vi "Periodic Tasks.vi"(8 "error in":errorcluster) -> ()   [LabVIEW 2018]
doc: "This VI runs in parallel to other tasks. It can contain as many user-defined periodic loops as you need. These can carry out PID or other sorts of timed response."
uses:
  LeftMotors.ctl
  RightMotors.ctl
  <vilib>/Rock Robotics/WPI/ThirdParty/Phoenix-LabVIEW/Motor Controller/Controls/CTRE_Phoenix_MotorControl_ControlMode.ctl
  Robot Global Data.vi
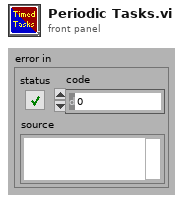
[diagram p1: front panel]
types:
  T1 = typedef "RightMotors.ctl" = enum16{"RightMotor1", "RightMotor2", "RightMotor3"}
  T2 = typedef "LeftMotors.ctl" = enum16{"LeftMotor1", "LeftMotor2", "LeftMotor3"}
  T3 = typedef "WPI_MotorControlDeviceRef.ctl" = cluster{"DeviceStatus":errorcluster, "Type":T4, "PWM":cluster{"PWM Channel":T5, "DeadBand":T6}, "CAN":cluster{"Device Number":u8, "SetOutput VI Ref":variant, "GetOutput VI Ref":variant, "Enable VI Ref":variant, "Disable VI Ref":variant, "Data":variant}, "Invert":bool, "DIO PWM":cluster{"PWM \"Enable\" Channel":T5, "DIOChannel":T7, "PWM Rate":dbl}}
  T4 = typedef "WPI_MotorControlType.ctl" = enum16{"PWM", "CAN", "DIO PWM"}
  T5 = typedef "FPGA_DIOPWMChannel.ctl" = enum8{"PWM 0", "PWM 1", "PWM 2", "PWM 3", "PWM 4", "PWM 5", "PWM 6", "PWM 7", "PWM 8", "PWM 9", "PWM MXP 0", "PWM MXP 1", "PWM MXP 2", "PWM MXP 3", "PWM MXP 4", "PWM MXP 5", "PWM MXP 6", "PWM MXP 7", "PWM MXP 8", "PWM MXP 9", "Invalid"}
  T6 = typedef "WPI_PWMDeadband.ctl" = cluster{"Name":string, "maxPositivePwm":i32, "minPositivePwm":i32, "centerPwm":i32, "maxNegativePwm":i32, "minNegativePwm":i32, "angularRange":u16}
  T7 = typedef "FPGA_DIOChannel.ctl" = enum8{"DIO 0", "DIO 1", "DIO 2", "DIO 3", "DIO 4", "DIO 5", "DIO 6", "DIO 7", "DIO 8", "DIO 9", "DIO MXP 0", "DIO MXP 1", "DIO MXP 2", "DIO MXP 3", "DIO MXP 4", "DIO MXP 5", "DIO MXP 6", "DIO MXP 7", "DIO MXP 8", "DIO MXP 9", "DIO MXP 10", "DIO MXP 11", "DIO MXP 12", "DIO MXP 13", "DIO MXP 14", "DIO MXP 15", "SPI Port CS1", "SPI Port CS2", "SPI Port CS3", "SPI Port MISO", "SPI Port MOSI", "Invalid"}
  T8 = typedef "CTRE_Phoenix_MotorControl_ControlMode.ctl" = u16
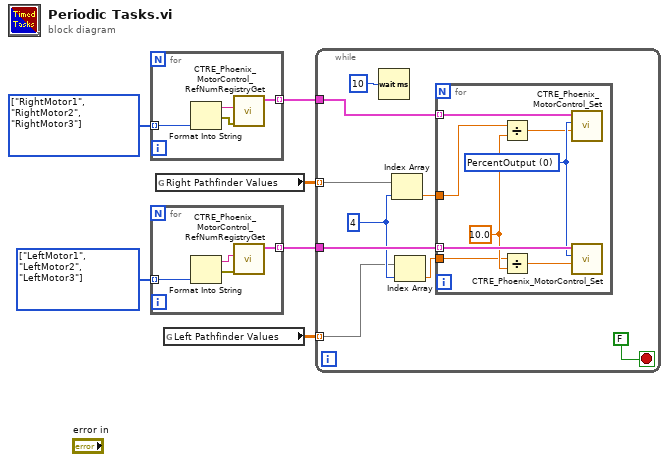
[diagram p0: block diagram]
diagram:
  w4 = T1[] [enum."RightMotor1", enum."RightMotor2", enum."RightMotor3"] items=["RightMotor1", "RightMotor2", "RightMotor3"] ("Array")
  w6 = T2[] [enum."LeftMotor1", enum."LeftMotor2", enum."LeftMotor3"] items=["LeftMotor1", "LeftMotor2", "LeftMotor3"] ("Array")
  n1 = for {
    tunnel: w4 -> [w9] mode=indexing
    tunnel: [w8] -> w3 mode=indexing
    n2 = Format Into String(w9) -> (resulting string=w10:string, error out=w7:errorcluster)  [unwired: 3 in]
    n3 = call <vilib>:"CTRE_Phoenix_MotorControl_RefNumRegistryGet.vi"("error in (no error)"=w7, "refnum name"=w10) -> ("PhoenixMotorControlDevRef"=w8:T3)  [unwired: 8 in, 1 out]
  }
  n4 = for {
    tunnel: w6 -> [w14] mode=indexing
    tunnel: [w12] -> w5 mode=indexing
    n5 = Format Into String(w14) -> (resulting string=w13:string, error out=w11:errorcluster)  [unwired: 3 in]
    n6 = call <vilib>:"CTRE_Phoenix_MotorControl_RefNumRegistryGet.vi"("error in (no error)"=w11, "refnum name"=w13) -> ("PhoenixMotorControlDevRef"=w12:T3)  [unwired: 8 in, 1 out]
  }
  n7 = global read "Robot Global Data.vi" "Right Pathfinder Values"() -> (w2:dbl[][])
  n8 = global read "Robot Global Data.vi" "Left Pathfinder Values"() -> (w1:dbl[][])
  n9 = while {
    tunnel: w5 -> [w23]
    tunnel: w3 -> [w22]
    tunnel: w2 -> [w16] mode=indexing
    tunnel: w1 -> [w15] mode=indexing
    stop <- FALSE stop-if-true
    w21 = 4 ("index")
    n10 = Wait (ms)(milliseconds to wait=u32 10) -> ()  [unwired: 1 out]
    n11 = Index Array(array=w16, index=w21) -> (element=w19:dbl)
    n12 = Index Array(array=w15, index=w21) -> (element=w20:dbl)
    n13 = for {
      tunnel: w23 -> [w31] mode=indexing
      tunnel: w22 -> [w30] mode=indexing
      tunnel: w20 -> [w25]
      tunnel: w19 -> [w24]
      w26 = 10.0 ("y")
      w29 = T8 0 items=["PercentOutput"=0, "Position"=1, "Velocity"=2, "Current"=3, "Follower"=5, "MotionProfile"=6, "MotionMagic"=7, "MotionProfileArc"=10, "Disabled"=15] ("Control Mode")
      n14 = Divide(x=w24, y=w26) -> (x/y=w27:dbl)
      n15 = Divide(x=w25, y=w26) -> (x/y=w28:dbl)
      n16 = call <vilib>:"CTRE_Phoenix_MotorControl_Set.vi"("Output"=w27, "Control Mode"=w29, "PhoenixMotorControlDevRef"=w30) -> ()  [unwired: 7 in, 2 out]
      n17 = call <vilib>:"CTRE_Phoenix_MotorControl_Set.vi"("Output"=w28, "Control Mode"=w29, "PhoenixMotorControlDevRef"=w31) -> ()  [unwired: 7 in, 2 out]
    }
  }
